vi "modbus output.vi"(8 "error in (no error)":errorcluster, 10 "data table in":T1, 11 "Modbus Module runtime in":refnum<class "Modbus Module runtime.lvclass">) -> (0 "error out":errorcluster, 2 "data table out":T1, 3 "Modbus Module runtime out":refnum<class "Modbus Module runtime.lvclass">)   [LabVIEW 2015, in "Modbus Module runtime.lvclass"]
uses:
  Modbus Module runtime.lvclass
  <vilib>/NI/Tag Bus/table/data table.ctl
  Modbus Module runtime.lvclass/Modbus Module runtime.ctl
  <vilib>/NI/Modbus Library/API/Slave/Modbus Slave.lvclass
  <vilib>/NI/Modbus Library/API/Modbus API.lvclass
  <vilib>/NI/Tag Bus/table/data table.lvlib
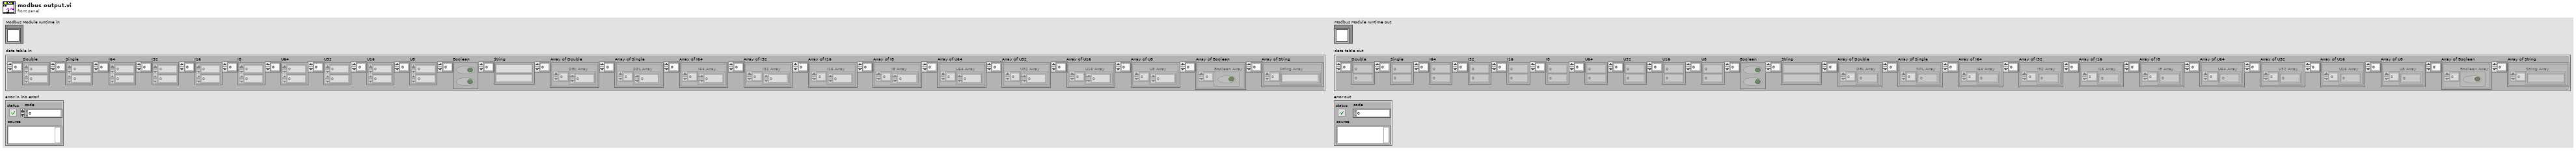
[diagram p1: front panel]
types:
  T1 = typedef "tag bus.lvlib/data table.lvlib/data table.ctl" = cluster{"Double":dbl[], "Single":sgl[], "I64":i64[], "I32":i32[], "I16":i16[], "I8":i8[], "U64":u64[], "U32":u32[], "U16":u16[], "U8":u8[], "Boolean":bool[], "String":string[], "Array of Double":cluster{"DBL Array":dbl[]}[], "Array of Single":cluster{"SGL Array":sgl[]}[], "Array of I64":cluster{"I64 Array":i64[]}[], "Array of I32":cluster{"I32 Array":i32[]}[], "Array of I16":cluster{"I16 Array":i16[]}[], "Array of I8":cluster{"I8 Array":i8[]}[], "Array of U64":cluster{"U64 Array":u64[]}[], "Array of U32":cluster{"U32 Array":u32[]}[], "Array of U16":cluster{"U16 Array":u16[]}[], "Array of U8":cluster{"U8 Array":u8[]}[], "Array of Boolean":cluster{"Boolean Array":bool[]}[], "Array of String":cluster{"String Array":string[]}[]}
  T2 = typedef "Modbus Module runtime.lvclass/output bulk data access.ctl" = cluster{"modbus type":T3, "start":u16, "length":u16, "maps":T4[], "coils":bool[], "registers":u16[]}
  T3 = typedef "Modbus Module Channel.lvclass/data bank type.ctl" = enum16{"Coils", "Discrete Inputs", "Input Registers", "Holding Registers"}
  T4 = typedef "Modbus Module runtime.lvclass/data mapping elements.ctl" = cluster{"data type":T5, "data index":i32, "element index":i32, "subindex/regcount":i32}
  T5 = typedef "tag bus.lvlib/tag descriptor.lvclass/Data Type.ctl" = enum16{"Double", "Single", "I64", "I32", "I16", "I8", "U64", "U32", "U16", "U8", "Boolean", "String", "Array of Double", "Array of Single", "Array of I64", "Array of I32", "Array of I16", "Array of I8", "Array of U64", "Array of U32", "Array of U16", "Array of U8", "Array of Boolean", "Array of String"}
  T6 = cluster{"32-bit: first word low":bool, "64-bit: first dword low":bool}
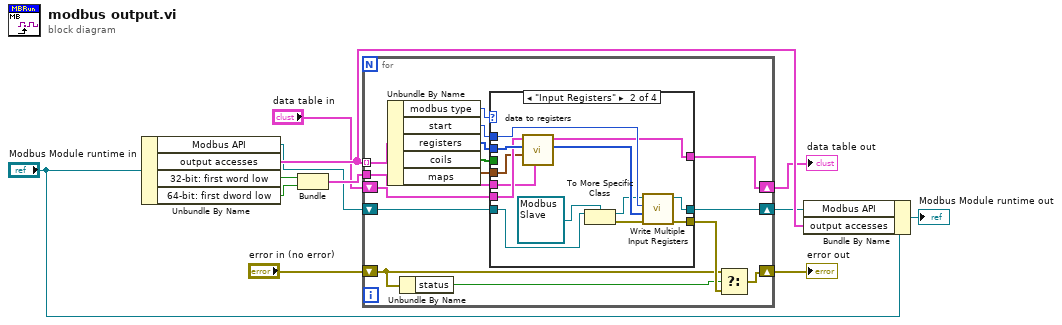
[diagram p0: block diagram]
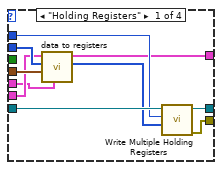
[diagram p2: hidden frame]
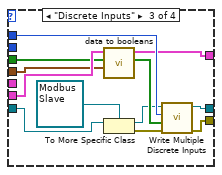
[diagram p3: hidden frame]
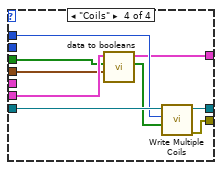
[diagram p4: hidden frame]
diagram:
  n1 = Unbundle By Name("Modbus Module runtime in") -> ("Modbus API"=w1:refnum<class "Modbus API.lvclass">, "output accesses"=w9:T2[], "32-bit: first word low"=w10:bool, "64-bit: first dword low"=w11:bool)
  n2 = Bundle("32-bit: first word low"=w10, "64-bit: first dword low"=w11) -> (w12:T6)  [unwired: 1 in]
  n3 = for {
    shift-right: [w24] -> w2
    shift-left: w1 -> [w25]
    shift-right: [w27] -> w8
    shift-left: "error in (no error)" -> [w15]
    tunnel: w9 -> [w26] mode=indexing
    shift-right: [w17] -> w5
    shift-left: "data table in" -> [w18]
    tunnel: w12 -> [w13]
    n4 = Unbundle By Name(w26) -> ("modbus type"=w22:T3, "start"=w21:u16, "registers"=w20:u16[], "coils"=w19:bool[], "maps"=w16:T4[])
    n5 = Unbundle By Name(w15) -> ("status"=w14:bool)
    n6 = case shown="\"Input Registers\"" w22 {
      tunnel: w25 -> [w37 w40 w52 w71]
      tunnel: [w36 w50 w62 w70] -> w24
      tunnel: [w34 w48 w60 w68] -> w23
      tunnel: w21 -> [w35 w49 w61 w69]
      tunnel: w20 -> [w33 w47 _ _]
      tunnel: w19 -> [_ _ w58 w65]
      tunnel: w18 -> [w31 w46 w59 w67]
      tunnel: [w30 w45 w57 w64] -> w17
      tunnel: w16 -> [w32 w43 w55 w66]
      tunnel: w13 -> [w28 w38 _ _]
      frame "Holding Registers" {
        n7 = call "data to registers.vi"("word order"=w28, "specifications"=w32, "allocation"=w33, "data table"=w31) -> ("registers"=w29:u16[], "allocation"=w30:T1)  [unwired: 6 in]
        n8 = call-dynamic "Write Multiple Holding Registers.vi"("registers to write"=w29, "starting address"=w35, "Modbus instance in"=w37) -> ("error out"=w34:errorcluster, "Modbus instance out"=w36:refnum<class "Modbus API.lvclass">)  [unwired: 7 in]
      }
      frame "Input Registers" {
        n9 = call "data to registers.vi"("word order"=w38, "specifications"=w43, "allocation"=w47, "data table"=w46) -> ("registers"=w44:u16[], "allocation"=w45:T1)  [unwired: 6 in]
        n10 = To More Specific Class(target class=refnum<class "Modbus Slave.lvclass"> refnum ("Modbus slave in"), reference=w40) -> (specific class reference=w41:refnum<class "Modbus Slave.lvclass">, error out=w39:errorcluster)  [unwired: 1 in]
        n11 = call-dynamic "Write Multiple Input Registers.vi"("error in"=w39, "input registers to write"=w44, "starting address"=w49, "Modbus slave in"=w41) -> ("error out"=w48:errorcluster, "Modbus slave out"=w50:refnum<class "Modbus Slave.lvclass">)  [unwired: 6 in]
      }
      frame "Discrete Inputs" {
        n12 = call "data to booleans.vi"("specifications"=w55, "allocation"=w58, "data table"=w59) -> ("registers"=w56:bool[], "allocation"=w57:T1)  [unwired: 7 in]
        n13 = To More Specific Class(target class=refnum<class "Modbus Slave.lvclass"> refnum ("Modbus slave in"), reference=w52) -> (specific class reference=w51:refnum<class "Modbus Slave.lvclass">, error out=w54:errorcluster)  [unwired: 1 in]
        n14 = call-dynamic "Write Multiple Discrete Inputs.vi"("error in"=w54, "discrete inputs to write"=w56, "starting address"=w61, "Modbus slave in"=w51) -> ("error out"=w60:errorcluster, "Modbus slave out"=w62:refnum<class "Modbus Slave.lvclass">)  [unwired: 6 in]
      }
      frame "Coils" {
        n15 = call "data to booleans.vi"("specifications"=w66, "allocation"=w65, "data table"=w67) -> ("registers"=w63:bool[], "allocation"=w64:T1)  [unwired: 7 in]
        n16 = call-dynamic "Write Multiple Coils.vi"("coils to write"=w63, "starting address"=w69, "Modbus instance in"=w71) -> ("error out"=w68:errorcluster, "Modbus instance out"=w70:refnum<class "Modbus API.lvclass">)  [unwired: 7 in]
      }
    }
    n17 = Select(t=w15, s=w14, f=w23) -> (s? t:f=w27:errorcluster)
  }
  "error out" <- w8
  "data table out" <- w5
  n18 = Bundle By Name(cluster="Modbus Module runtime in", "Modbus API"=w2, "output accesses"=w9) -> (→"Modbus Module runtime out":refnum<class "Modbus Module runtime.lvclass">)
